vi "Change Tile Type If Matches.vi"(8 "Change To":T1, 9 "Initial Type":T1, 10 "Array Indices":cluster{i32, i32}, 11 "Board in":T1[][](array[typedef])) -> (2 "Matched Initial Type":bool, 3 "Board out":T1[][](array[typedef]))   [LabVIEW 2019]
uses:
  Tile State.ctl
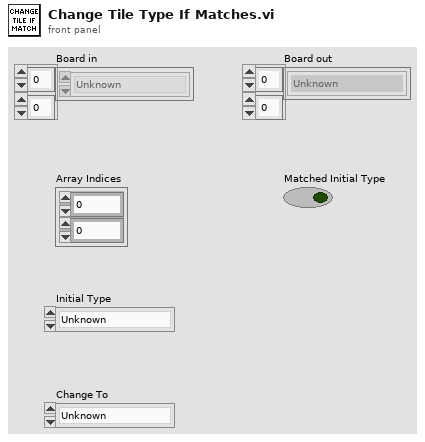
[diagram p1: front panel]
types:
  T1 = typedef "Tile State.ctl" = enum16{"Unknown", "Empty Water", "My Ship (Hidden)", "My Ship (Hit)", "Opponent's Ship (Revealed)", "Oponnent's Ship (Hit)", "Tentative Location"}
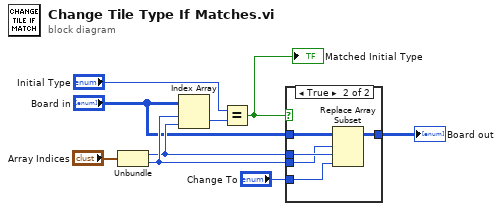
[diagram p0: block diagram]
diagram:
  n1 = Unbundle("Array Indices") -> (w8:i32, w9:i32)
  n2 = Index Array(array="Board in", index (row)=w9, index (col)=w8) -> (element=w5:T1)
  n3 = Equal?(x="Initial Type", y=w5) -> (x = y?=w7:bool)
  "Matched Initial Type" <- w7
  n4 = case shown="True" w7 {
    tunnel: [w10 w15] -> w3
    tunnel: "Board in" -> [w10 w14]
    tunnel: w8 -> [_ w13]
    tunnel: w9 -> [_ w12]
    tunnel: "Change To" -> [_ w11]
    frame False {
    }
    frame True {
      n5 = Replace Array Subset(array=w14, new element=w11, index (row)=w12, index (col)=w13) -> (w15:T1[][])
    }
  }
  "Board out" <- w3
